vi "solar_qtimer Release.vi"(6 "Suppress Errors? (T)":bool=TRUE, 8 "error in (no error)":errorcluster, 10 "Force Destroy? (F)":bool, 11 "QTimer Refnum":T4) -> (0 "error out":errorcluster, 3 "QTimer":T1)   [LabVIEW 2018]
doc: "This releases the QTimer reference."
uses:
  solar_qtimer_ctl Refnum.ctl
  solar_qtimer_ctl QTimer.ctl
  solar_qtimer_ctl SEQ.ctl
  solar_qtimer_ctl QTimer Settings.ctl
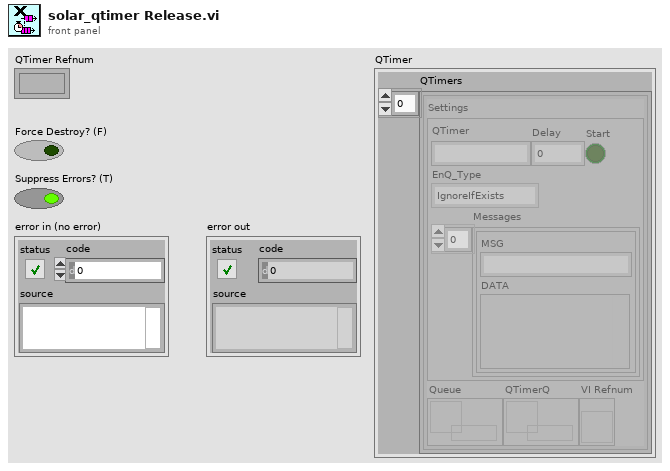
[diagram p1: front panel]
types:
  T1 = typedef "solar_qtimer_ctl SEQ.ctl" = cluster{"QTimers":T2[]}
  T2 = typedef "solar_qtimer_ctl QTimer.ctl" = cluster{"Settings":T3, "Queue":refnum<queue>, "QTimerQ":refnum<queue>, "VI Refnum":refnum<vi>}
  T3 = typedef "solar_qtimer_ctl QTimer Settings.ctl" = cluster{"QTimer":string, "Delay":i32, "Start":bool, "EnQ_Type":enum8{"Normal", "Priority", "IgnoreIfExists"}, "Messages":cluster{"MSG":string, "DATA":variant}[]}
  T4 = typedef "solar_qtimer_ctl Refnum.ctl" = refnum<k1>
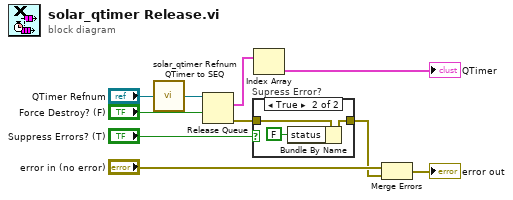
[diagram p0: block diagram]
diagram:
  n1 = call "solar_qtimer Refnum QTimer to SEQ.vi"("QTimer Refnum"="QTimer Refnum") -> ("QTimers SEQ"=w7:refnum<queue>)
  n2 = Release Queue(queue=w7, force destroy? (F)="Force Destroy? (F)") -> (remaining elements=w5:T1[], error out=w2:errorcluster)  [unwired: 1 in, 1 out]
  n3 = case "Supress Error?" shown="True" "Suppress Errors? (T)" {
    tunnel: w2 -> [w11 w14]
    tunnel: [w11 w12] -> w1
    frame False {
    }
    frame True {
      n4 = Bundle By Name(cluster=w14, "status"=FALSE) -> (w12:errorcluster)
    }
  }
  n5 = Index Array(array=w5) -> (element=→"QTimer":T1)  [unwired: 1 in]
  n6 = Merge Errors("error in (no error)", w1) -> (→"error out":errorcluster)
